vi "TCP Listener.vi"() -> ()   [LabVIEW 2019]
panel:
  out "No of messages":i32
  out "Recieved Messages":string[](array[string])
  out "Current Message":string
  in  "error in (no error)":errorcluster
  out "error out":errorcluster
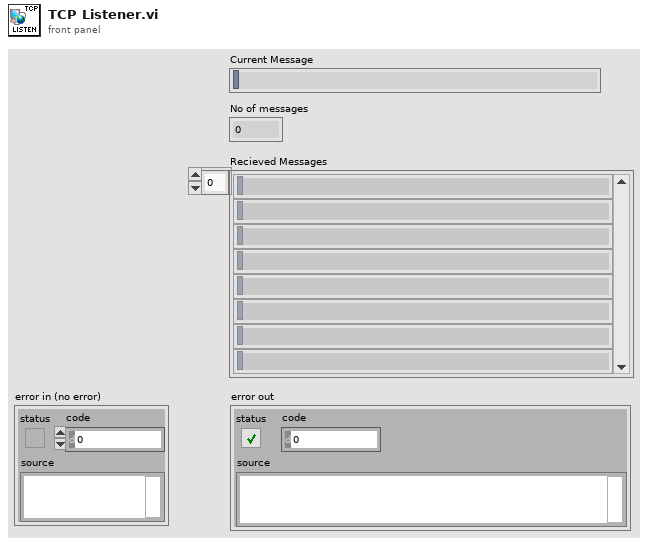
[diagram p1: front panel]
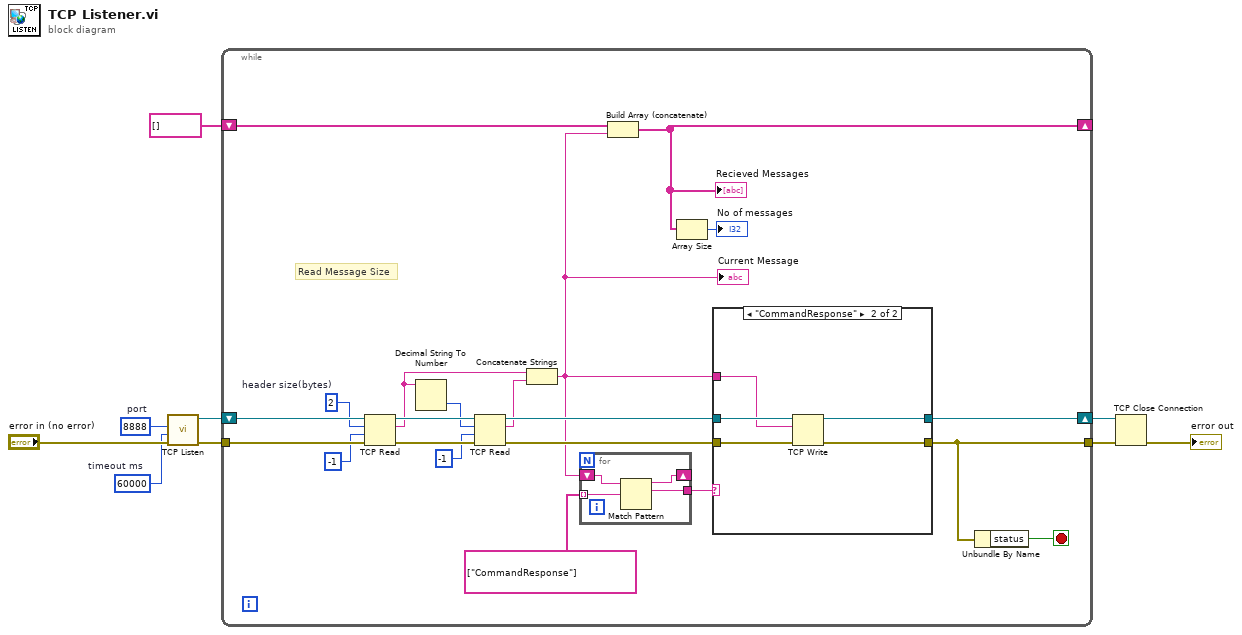
[diagram p0: block diagram]
diagram:
  w1 = 60000  # timeout ms
  w6 = u16 8888  # port
  n1 = call <vilib>:"TCP Listen.vi"("error in (no error)"="error in (no error)", "timeout ms (wait forever: -1)"=w1, "port"=w6) -> ("error out"=w4:errorcluster, "connection ID"=w5:refnum<k5>)  [unwired: 4 in, 3 out]
  n2 = while {
    shift-right: [w15] -> _
    shift-left: string[] [] -> [w28]
    shift-right: [w17] -> w9
    shift-left: w5 -> [w30]
    tunnel: w4 -> [w29]
    tunnel: [w19] -> w8
    stop <- w20 stop-if-true
    w27 = 2  # header size(bytes)
    # "Read Message Size"
    n3 = TCP Read(connection ID=w30, bytes to read=w27, error in (no error)=w29, 9:-1 ("timeout ms (25000)")) -> (connection ID out=w24:refnum<k5>, data out=w10:string, error out=w25:errorcluster)  [unwired: 1 in]
    n4 = Decimal String To Number(string=w10) -> (number=w23:i32)  [unwired: 2 in, 1 out]
    n5 = TCP Read(connection ID=w24, bytes to read=w23, error in (no error)=w25, 9:-1 ("timeout ms (25000)")) -> (connection ID out=w18:refnum<k5>, data out=w12:string, error out=w21:errorcluster)  [unwired: 1 in]
    n6 = Concatenate Strings(w10, w12) -> (w11:string)
    "Current Message" <- w11
    n7 = for {
      tunnel: string[] ["CommandResponse"] ("regular expression") -> [w33] mode=indexing
      tunnel: [w34] -> w14
      shift-right: [w31] -> _
      shift-left: w11 -> [w32]
      n8 = Match Pattern(string=w32, regular expression=w33) -> (before substring=w31:string, match substring=w34:string)  [unwired: 1 in, 2 out]
    }
    n9 = Build Array (concatenate)(w28, w11) -> (w15:string[])
    "Recieved Messages" <- w15
    n10 = Array Size(array=w15) -> (size(s)=→"No of messages":i32)
    n11 = case shown="\"CommandResponse\"" w14 {
      tunnel: w21 -> [w36 w41]
      tunnel: [w36 w40] -> w19
      tunnel: w18 -> [w35 w39]
      tunnel: [w35 w38] -> w17
      tunnel: w11 -> [_ w37]
      frame "CommandOnly", Default {
      }
      frame "CommandResponse" {
        n12 = TCP Write(connection ID=w39, data in=w37, error in (no error)=w41) -> (connection ID out=w38:refnum<k5>, error out=w40:errorcluster)  [unwired: 1 in, 1 out]
      }
    }
    n13 = Unbundle By Name(w19) -> ("status"=w20:bool)
  }
  n14 = TCP Close Connection(connection ID=w9, error in (no error)=w8) -> (error out=→"error out":errorcluster)  [unwired: 1 in, 1 out]
